vi "Write File Data Msg.vi"(9 "File Data Msg":refnum<class "File Data Msg.lvclass">, 11 "Open File in":refnum<class "Open File.lvclass">) -> (3 "Open File out":refnum<class "Open File.lvclass">)   [LabVIEW 2018, in "Open File Actor.lvlib" / "Open File.lvclass"]
uses:
  Open File.lvclass
  Open File Messages/File Data Msg/File Data Msg.lvclass
  Open File.lvclass/Open File.ctl
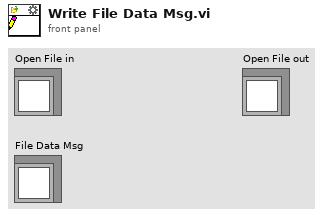
[diagram p1: front panel]
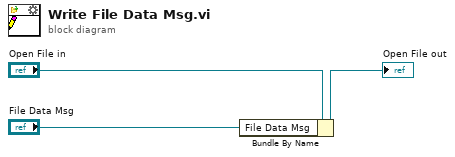
[diagram p0: block diagram]
diagram:
  n1 = Bundle By Name(cluster="Open File in", "File Data Msg"="File Data Msg") -> (→"Open File out":refnum<class "Open File.lvclass">)
